vi "fcs_add.vi"(0 "Array in":sgl[][](array[numeric]), 1 "byte offset in":i64, 2 "Path in":path, 3 "error in (no error)":errorcluster) -> (6 "total data":sgl[][](array[numeric]), 7 "new data":sgl[][](array[numeric]), 8 "byte offset out":i64, 9 "error out":errorcluster)   [LabVIEW 2013]
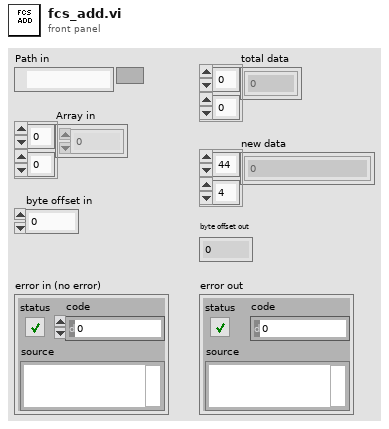
[diagram p1: front panel]
types:
  T1 = enum16{"big-endian, network order", "native, host order", "little-endian"}
  T2 = enum16{"open", "replace", "create", "open or create", "replace or create", "replace or create with confirmation"}
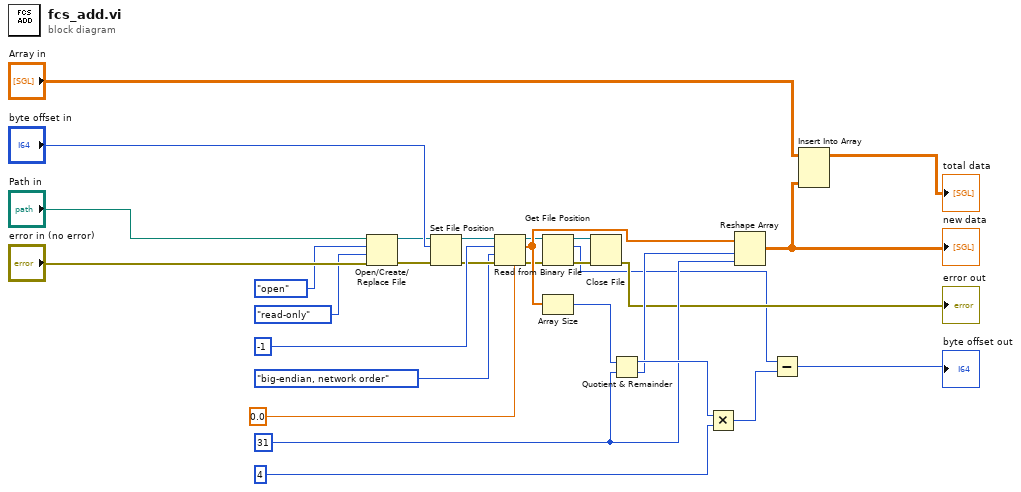
[diagram p0: block diagram]
diagram:
  w18 = 31 ("dimension size")
  n1 = Open/Create/Replace File(file path (use dialog)="Path in", error in="error in (no error)", operation (0:open)=T2."open", access (0:read/write)=enum16{"read/write", "read-only", "write-only"}."read-only") -> (refnum out=w8:refnum<file>, error out=w11:errorcluster)  [unwired: 2 in, 1 out]
  n2 = Set File Position(offset (in bytes) (0)="byte offset in", refnum=w8, error in=w11) -> (refnum out=w9:refnum<file>, error out=w10:errorcluster)  [unwired: 1 in]
  n3 = Read from Binary File(5:sgl 0.0, 8:w10, 9:T1."big-endian, network order" ("byte order (0:big-endian, network order)"), 10:-1, 11:w9) -> (0:w12:errorcluster, 2:w17:sgl[], 3:w14:refnum<file>)  [unwired: 1 in, 1 out]
  n4 = Get File Position(4:w12, 7:w14) -> (0:w13:errorcluster, 2:w1:i64, 3:w15:refnum<file>)
  n5 = Array Size(array=w17) -> (size(s)=w19:i32)
  n6 = Close File(refnum=w15, error in=w13) -> (error out=→"error out":errorcluster)  [unwired: 1 out]
  n7 = Quotient & Remainder(x=w19, y=w18) -> (x-y*floor(x/y)=w22:i32, floor(x/y)=w20:i32)
  n8 = Multiply(x=w22, y=4) -> (x*y=w23:i32)
  n9 = Reshape Array(w17, w20, w18) -> (w29:sgl[][])
  "new data" <- w29
  n10 = Subtract(x=w1, y=w23) -> (x-y=→"byte offset out":i64)
  n11 = Insert Into Array(array="Array in", new element=w29) -> (→"total data":sgl[][])  [unwired: 2 in]
